vi "[FGV]Parameters.vi"(7 "Parameter":T2, 8 "Error In":errorcluster, 9 "ParameterData In":T1, 10 "ParamName":string, 11 "Parameter":variant) -> (0 "Error Out":errorcluster, 3 "ParameterData Out":T1)   [LabVIEW 2019]
uses:
  Controls/Parameter.ctl
  Controls/ParameterData.ctl
  558e01b3-27a1-429a-ad60-d0add2b8f394.vi
  ca725f02-9438-4a56-9ae5-b8e7613ce0a2.vi
  LLB/Commonly VI/Main Glb.vi
  <vilib>/JDP Science/JSONtext/Variant to JSON Text.vi
  <vilib>/JDP Science/JSONtext/JSON text to Variant.vi
  LLB/Commonly VI.lvlib
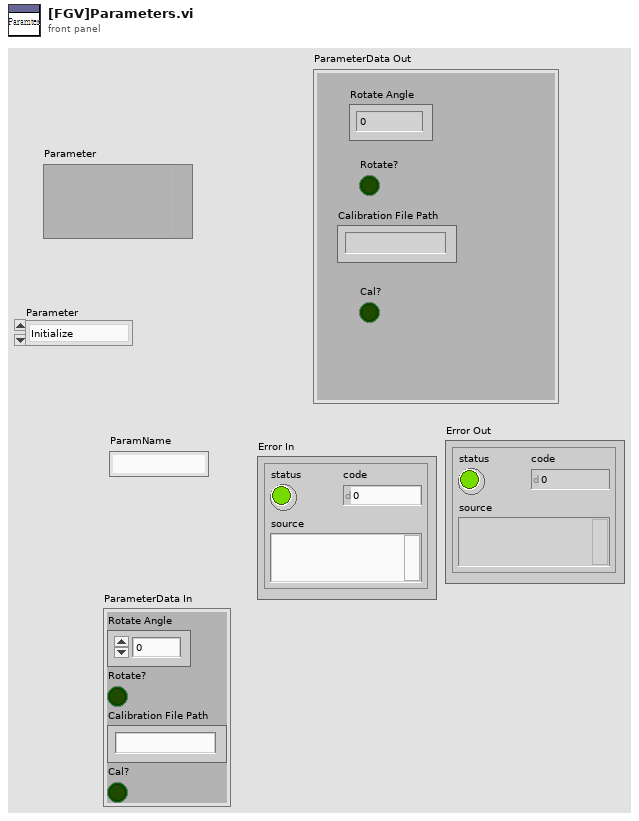
[diagram p1: front panel]
types:
  T1 = typedef "ParameterData.ctl" = cluster{"Rotate Angle":dbl, "Rotate?":bool, "Calibration File Path":string, "Cal?":bool}
  T2 = typedef "Parameter.ctl" = enum16{"Initialize", "Write", "Read", "WriteAll", "Save", "Load"}
  T3 = typedef "Image Type" = u32
  T4 = typedef "IMAQ Image.ctl" = refnum<image>
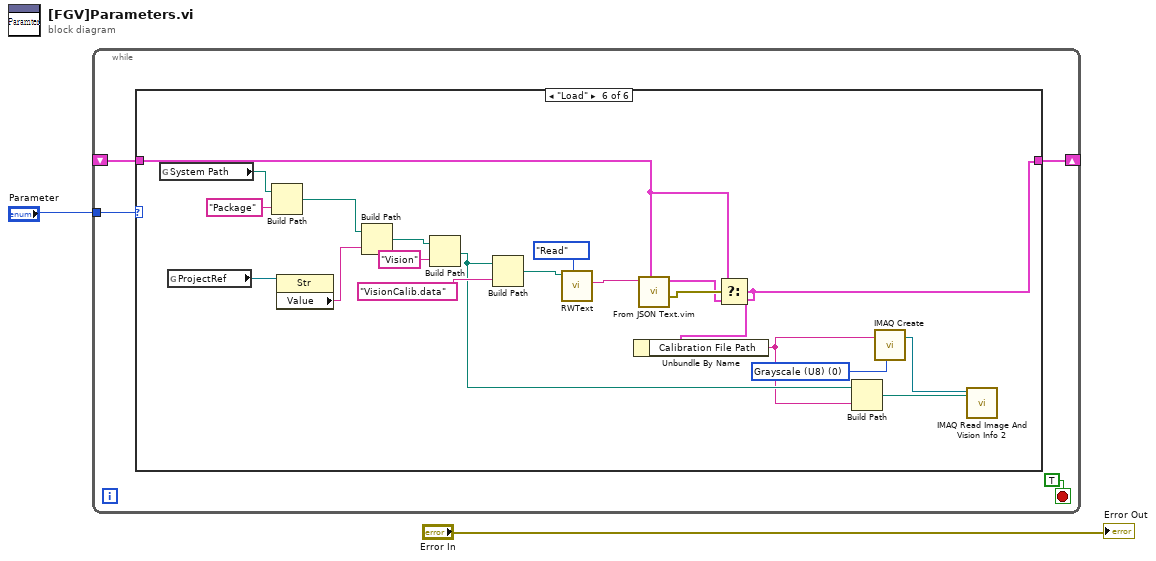
[diagram p0: block diagram]
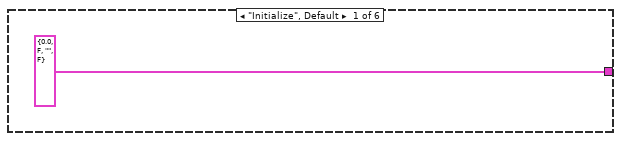
[diagram p2: hidden frame]
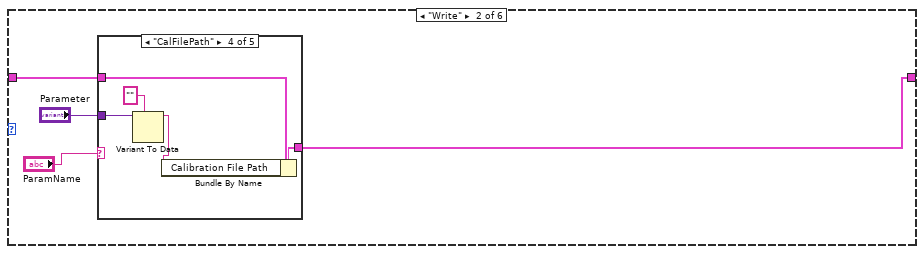
[diagram p3: hidden frame]
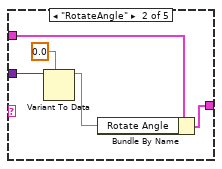
[diagram p5: hidden frame]
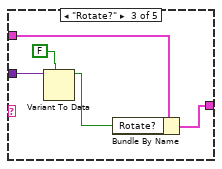
[diagram p6: hidden frame]
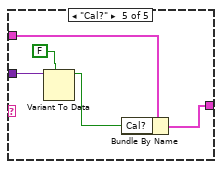
[diagram p7: hidden frame]
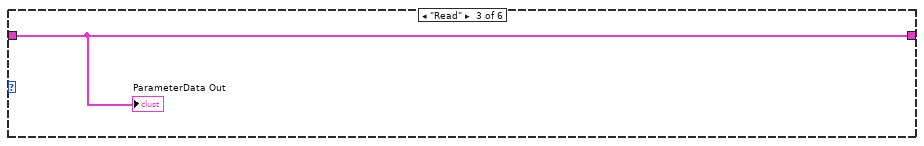
[diagram p8: hidden frame]
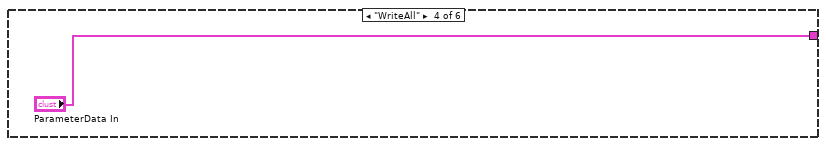
[diagram p9: hidden frame]
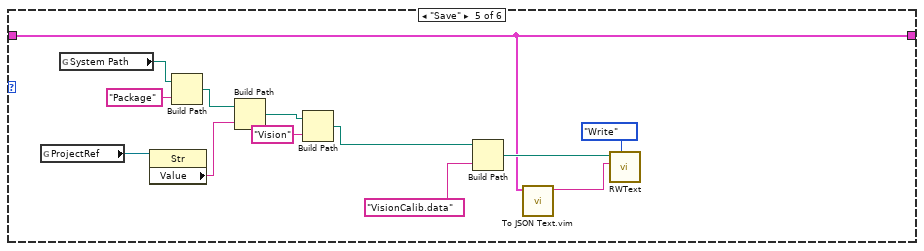
[diagram p10: hidden frame]
diagram:
  n1 = while {
    tunnel: "Parameter" -> [w5]
    shift-right: [w4] -> _
    shift-left: _ -> [w3]
    stop <- TRUE ("stop") stop-if-true
    n2 = case shown="\"Load\"" w5 {
      tunnel: [T1 {"Rotate Angle"=0.0, "Rotate?"=FALSE, "Calibration File Path"="", "Cal?"=FALSE} ("ParameterData In") w10 w33 "ParameterData In" w40 w52] -> w4
      tunnel: w3 -> [_ w11 w33 _ w40 w58]
      frame "Initialize", Default {
      }
      frame "Write" {
        n3 = case shown="\"CalFilePath\"" "ParamName" {
          tunnel: w11 -> [w12 w17 w22 w27 w32]
          tunnel: [w12 w16 w21 w26 w31] -> w10
          tunnel: "Parameter" -> [_ w15 w20 w25 w30]
          frame "False", Default {
          }
          frame "RotateAngle" {
            n4 = Variant To Data(type=0.0 ("Rotate Angel"), Variant=w15) -> (data=w13:dbl)  [unwired: 1 in, 1 out]
            n5 = Bundle By Name(cluster=w17, "Rotate Angle"=w13) -> (w16:T1)
          }
          frame "Rotate?" {
            n6 = Variant To Data(type=FALSE, Variant=w20) -> (data=w19:bool)  [unwired: 1 in, 1 out]
            n7 = Bundle By Name(cluster=w22, "Rotate?"=w19) -> (w21:T1)
          }
          frame "CalFilePath" {
            n8 = Variant To Data(type="" ("Calibration File Path"), Variant=w25) -> (data=w23:string)  [unwired: 1 in, 1 out]
            n9 = Bundle By Name(cluster=w27, "Calibration File Path"=w23) -> (w26:T1)
          }
          frame "Cal?" {
            n10 = Variant To Data(type=FALSE, Variant=w30) -> (data=w29:bool)  [unwired: 1 in, 1 out]
            n11 = Bundle By Name(cluster=w32, "Cal?"=w29) -> (w31:T1)
          }
        }
      }
      frame "Read" {
        "ParameterData Out" <- w33
      }
      frame "WriteAll" {
      }
      frame "Save" {
        n12 = global read "Main Glb.vi" "ProjectRef"() -> (w47:refnum<vi>)
        n13 = global read "Main Glb.vi" "System Path"() -> (w38:path)
        n14 = property class="Str"(reference=w47) -> ("Value"=w46:string)  [unwired: 1 in, 2 out]
        n15 = Build Path(base path=w38, name or relative path="Package") -> (appended path=w36:path)
        n16 = Build Path(base path=w36, name or relative path=w46) -> (appended path=w45:path)
        n17 = Build Path(base path=w45, name or relative path="Vision") -> (appended path=w35:path)
        n18 = Build Path(base path=w35, name or relative path="VisionCalib.data") -> (appended path=w42:path)
        n19 = call "To JSON Text.vim"("Anything"=w40) -> ("<JSON>"=w39:string)  [unwired: 9 in, 1 out]
        n20 = call "RWText.vi"("Action"=enum16{"Read", "Write"}."Write", "TextIn"=w39, "file path (use dialog)"=w42) -> ()  [unwired: 7 in, 2 out]
      }
      frame "Load" {
        w48 = T3 0 items=["Grayscale (U8)", "Grayscale (I16)", "Grayscale (SGL)", "Complex (CSG)", "RGB (U32)", "HSL (U32)", "RGB (U64)", "Grayscale (U16)"] ("Image Type")
        n21 = global read "Main Glb.vi" "System Path"() -> (w55:path)
        n22 = global read "Main Glb.vi" "ProjectRef"() -> (w67:refnum<vi>)
        n23 = Build Path(base path=w55, name or relative path="Package") -> (appended path=w56:path)
        n24 = property class="Str"(reference=w67) -> ("Value"=w66:string)  [unwired: 1 in, 2 out]
        n25 = Build Path(base path=w56, name or relative path=w66) -> (appended path=w65:path)
        n26 = Build Path(base path=w65, name or relative path="Vision") -> (appended path=w57:path)
        n27 = Build Path(base path=w57, name or relative path="VisionCalib.data") -> (appended path=w62:path)
        n28 = call "RWText.vi"("Action"=enum16{"Read", "Write"}."Read", "file path (use dialog)"=w62) -> ("textOut"=w53:string)  [unwired: 8 in, 1 out]
        n29 = call "From JSON Text.vim"("Data Type and Default Value"=w58, "JSON"=w53) -> ("error out"=w60:errorcluster, "Data out"=w59:T1)  [unwired: 8 in]
        n30 = Select(t=w58, s=w60, f=w59) -> (s? t:f=w52:T1)
        n31 = Unbundle By Name(w52) -> ("Calibration File Path"=w49:string)
        n32 = Build Path(base path=w57, name or relative path=w49) -> (appended path=w51:path)
        n33 = call "IMAQ Create"("Image Name"=w49, "Image Type"=w48) -> ("New Image"=w50:T4)  [unwired: 3 in, 1 out]
        n34 = call "IMAQ Read Image And Vision Info 2"("File Path"=w51, "Image"=w50) -> ()  [unwired: 7 in, 3 out]
      }
    }
  }
  "Error Out" <- "Error In"
